vi "Write Connection Configuration.vi"(8 "error in (no error)":errorcluster, 10 "Connection Configuration":refnum<class "Connection.lvclass">, 11 "MQTT_Base in":refnum<class "MQTT_Base.lvclass">) -> (0 "error out":errorcluster, 3 "MQTT_Base out":refnum<class "MQTT_Base.lvclass">)   [LabVIEW 2013, in "MQTT Base.lvlib" / "MQTT_Base.lvclass"]
uses:
  MQTT_Base.lvclass
  MQTT_Connection/Connection/Connection.lvclass
  MQTT_Base.lvclass/MQTT_Base.ctl
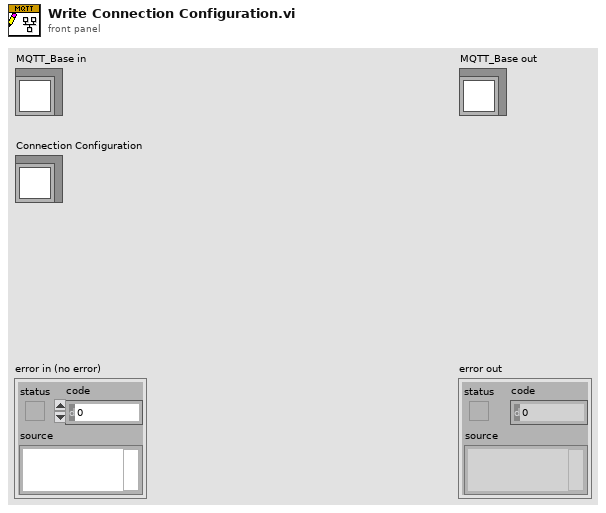
[diagram p1: front panel]
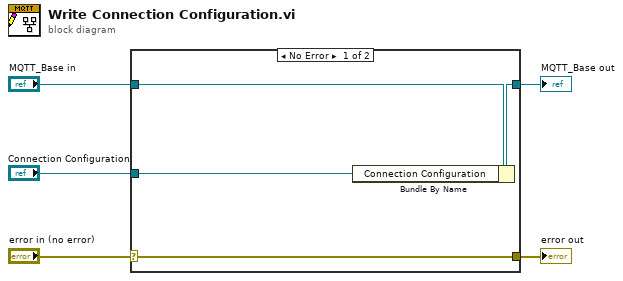
[diagram p0: block diagram]
diagram:
  n1 = case shown="No Error" "error in (no error)" {
    selector: "error in (no error)" -> [w9 w10]
    tunnel: [w9 w10] -> w4
    tunnel: [w7 w11] -> w2
    tunnel: "MQTT_Base in" -> [w8 w11]
    tunnel: "Connection Configuration" -> [w6 _]
    frame No Error {
      n2 = Bundle By Name(cluster=w8, "Connection Configuration"=w6) -> (w7:refnum<class "MQTT_Base.lvclass">)
    }
    frame Error {
    }
  }
  "error out" <- w4
  "MQTT_Base out" <- w2
